vi "MyOrdinaryClass_Create.vi"(0 "reference in":refnum<class "MyOrdinaryClass.lvclass">, 5 "error in (no error)":errorcluster) -> (14 "reference out":refnum<class "MyOrdinaryClass.lvclass">, 19 "error out":errorcluster)   [LabVIEW 2017, in "MyOrdinaryClass.lvclass"]
doc: "Constructor."
uses:
  MyOrdinaryClass.lvclass
  C:/Program Files/National Instruments/LabVIEW 2017/vi.lib/addons/_AddQ/G#Object/G#Object.lvclass
  <vilib>/addons/_AddQ/G#Object/G#Object.lvclass
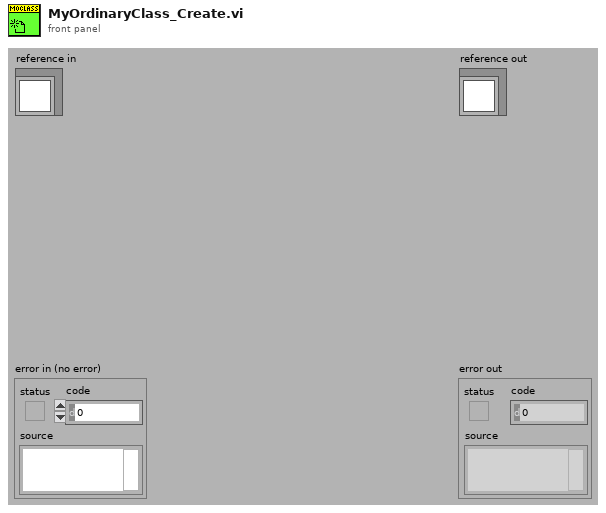
[diagram p1: front panel]
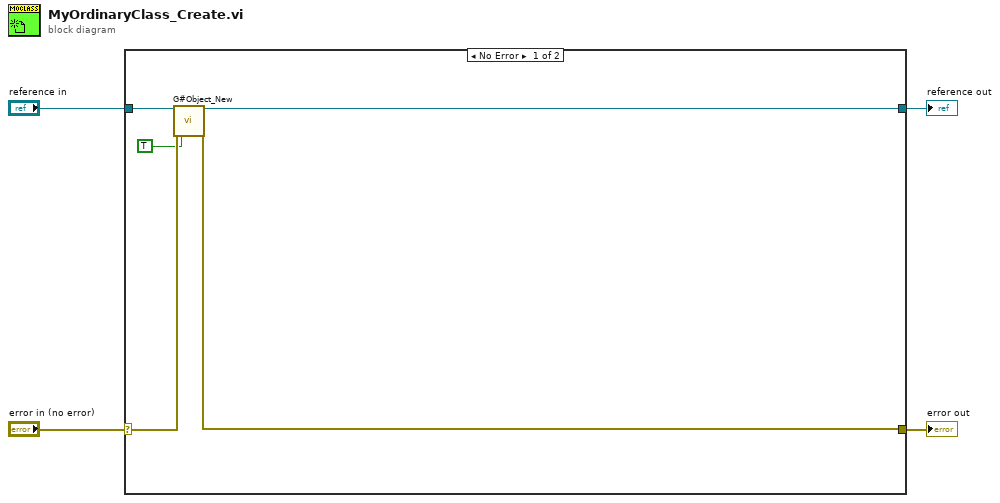
[diagram p0: block diagram]
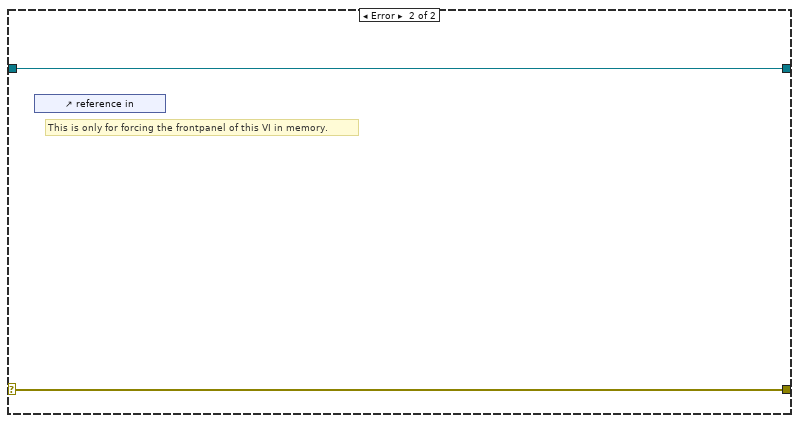
[diagram p2: hidden frame]
diagram:
  n1 = case shown="No Error" "error in (no error)" {
    selector: "error in (no error)" -> [w8 w11]
    tunnel: [w5 w11] -> w3
    tunnel: [w6 w10] -> w1
    tunnel: "reference in" -> [w9 w10]
    frame No Error {
      n2 = call <vilib>:"G#Object_New.vi"("reference in"=w9, "error in (no error)"=w8, "user counter (T)?"=TRUE ("User Counter")) -> ("reference out"=w6:refnum<class "MyOrdinaryClass.lvclass">, "error out"=w5:errorcluster)  [unwired: 14 in, 1 out]
    }
    frame Error {
      # "This is only for forcing the frontpanel of this VI in memory."
      n3 = control-ref of="reference in"() -> ()  [unwired: 1 out]
    }
  }
  "error out" <- w3
  "reference out" <- w1
